vi "deinitialize.vi"(0 "HGF_DSCVarManager":refnum<class "HGF_DSCVarManager.lvclass">, 5 "error in (no error)":errorcluster) -> (19 "error out":errorcluster)   [LabVIEW 2012, in "HGF_DSC.lvlib" / "HGF_DSCVarManager.lvclass"]
doc: "This is a dynamic dispatch VI. It can be overwritten by childclasses to release allocated recources."
uses:
  HGF_DSCVarManager.lvclass
  HGF_BaseClasses/HGF_Visitable/HGF_Visitable.lvclass
  HGF_DSCVarManager.lvclass/HGF_DSCVarManager.ctl
  <vilib>/lvdsc/NI_DSC.lvlib
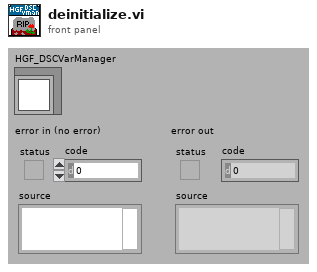
[diagram p1: front panel]
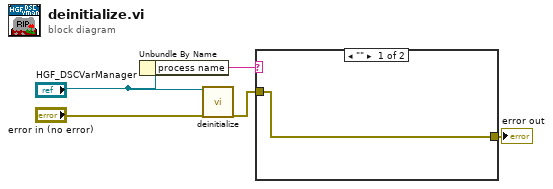
[diagram p0: block diagram]
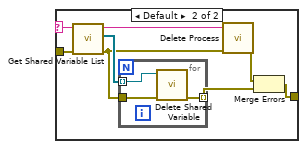
[diagram p2: hidden frame]
diagram:
  n1 = Unbundle By Name("HGF_DSCVarManager") -> ("process name"=w1:string)
  n2 = call-parent "deinitialize.vi"("HGF_Factory"="HGF_DSCVarManager", "error in (no error)"="error in (no error)") -> ("error out"=w3:errorcluster)  [unwired: 17 out]
  n3 = case shown="\"\"" w1 {
    selector: w1 -> [_ w7]
    tunnel: w3 -> [w6 w14]
    tunnel: [w6 w8] -> w2
    frame "" {
    }
    frame Default {
      n4 = call <vilib>:"Get Shared Variable List.vi"("error in (no error)"=w14, "process name"=w7) -> ("error out"=w11:errorcluster, "shared variables"=w13:refnum<k21>[], "process name out"=w12:string)  [unwired: 7 out]
      n5 = for {
        tunnel: w13 -> [w17] mode=indexing
        tunnel: w11 -> [w16]
        tunnel: [w15] -> w9 mode=indexing
        n6 = call <vilib>:"Delete Shared Variable.vi"("error in (no error)"=w16, "shared variable"=w17) -> ("error out"=w15:errorcluster)  [unwired: 9 out]
      }
      n7 = call <vilib>:"Delete Process.vi"("error in (no error)"=w11, "process name"=w12) -> ("error out"=w10:errorcluster)  [unwired: 9 out]
      n8 = Merge Errors(w10, w9) -> (w8:errorcluster)
    }
  }
  "error out" <- w2
